vi "Configure Multi Eval Meas Limit SEM Test Tolerance.vi"(6 "Tolerance 6 GHz (0.0)":dbl format="%^.3e", 7 "Tolerance 4 GHz (0.0)":dbl format="%^.3e", 8 "error in (no error)":errorcluster, 9 "Tolerance 3 GHz (0.0)":dbl format="%^.3e", 10 "Instance (1)":T1=1, 11 "VISA resource name":refnum<visa-resource-name>) -> (0 "error out":errorcluster, 3 "VISA resource name out":refnum<visa-resource-name>)   [LabVIEW 2020, in "Rohde&Schwarz CMWXP NR FR1 Measurement.lvlib"]
doc: "Defines the test tolerance for spectrum emission masks, depending on the carrier frequency.\n\nAttribute:\nRSCMWXPNRFR1M_ATTR_MULTI_EVAL_MEAS_LIMIT_SEM_TEST_TOLERANCE\n\nRemote-control command:\nCONFigure:NRSub:MEAS<i>:MEValuation:LIMit:SEMask:TTOLerance"
uses:
  <instrlib>/Rohde&Schwarz CMWXP NR FR1 Measurement/Rohde&Schwarz CMWXP NR FR1 Measurement.lvlib
  <instrlib>/Rohde&Schwarz CMWXP NR FR1 Measurement/Private/_Instance.ctl
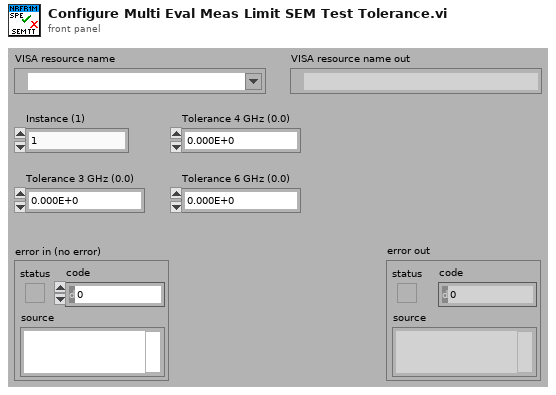
[diagram p1: front panel]
types:
  T1 = typedef "Rohde&Schwarz CMWXP NR FR1 Measurement.lvlib/_Instance.ctl" = i32
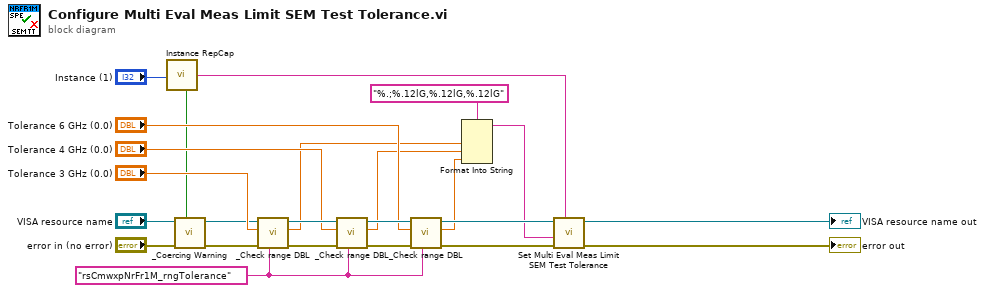
[diagram p0: block diagram]
diagram:
  w11 = "rsCmwxpNrFr1M_rngTolerance" ("Range Table Identifier")
  n1 = call <instrlib>:"Instance RepCap.vi"("Instance In"="Instance (1)") -> ("In Range?"=w1:bool, "RepCap Identifier Out"=w21:string)  [unwired: 1 in]
  n2 = call <instrlib>:"_Coercing Warning.vi"("In Range?"=w1, "error in (no error)"="error in (no error)", "VISA resource name"="VISA resource name") -> ("error out"=w3:errorcluster, "VISA resource name out"=w2:refnum<visa-resource-name>)  [unwired: 7 in]
  n3 = call <instrlib>:"_Check range DBL.vi"("Range Table Identifier"=w11, "error in (no error)"=w3, "DBL Value In"="Tolerance 3 GHz (0.0)", "VISA resource name"=w2) -> ("error out"=w19:errorcluster, "DBL Value Out"=w9:dbl, "VISA resource name out"=w18:refnum<visa-resource-name>)  [unwired: 5 in]
  n4 = call <instrlib>:"_Check range DBL.vi"("Range Table Identifier"=w11, "error in (no error)"=w19, "DBL Value In"="Tolerance 4 GHz (0.0)", "VISA resource name"=w18) -> ("error out"=w17:errorcluster, "DBL Value Out"=w8:dbl, "VISA resource name out"=w16:refnum<visa-resource-name>)  [unwired: 5 in]
  n5 = call <instrlib>:"_Check range DBL.vi"("Range Table Identifier"=w11, "error in (no error)"=w17, "DBL Value In"="Tolerance 6 GHz (0.0)", "VISA resource name"=w16) -> ("error out"=w15:errorcluster, "DBL Value Out"=w7:dbl, "VISA resource name out"=w14:refnum<visa-resource-name>)  [unwired: 5 in]
  n6 = Format Into String(format string="%.;%.12lG,%.12lG,%.12lG", w9, w8, w7) -> (resulting string=w6:string)  [unwired: 2 in, 1 out]
  n7 = call "Set Multi Eval Meas Limit SEM Test Tolerance"("Repeated Capabilities"=w21, "error in (no error)"=w15, "Multi Eval Meas Limit SEM Test Tolerance ()"=w6, "instrument handle"=w14) -> ("error out"=→"error out":errorcluster, "instrument handle out"=→"VISA resource name out":refnum<visa-resource-name>)  [unwired: 6 in]
